vi "SubPanel_Size and Insert.vi"(6 "Border Spacing":i32=-2, 7 "VI":refnum<vi>, 8 "Error":errorcluster, 9 "Frame Ref":refnum<vi>, 10 "Lock Subpanel Size":bool, 11 "Sub Panel":refnum<vi>) -> (0 "Error Out":errorcluster, 1 "Vi Inserted Out":bool, 2 "Success Out":bool, 3 "Sub Panel Out":refnum<vi>)   [LabVIEW 2020]
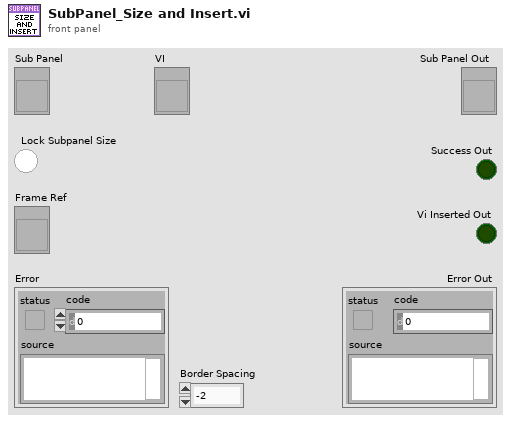
[diagram p1: front panel]
types:
  T1 = typedef "LVRectTypeDef.ctl" = cluster{"Left":i16, "Top":i16, "Right":i16, "Bottom":i16}
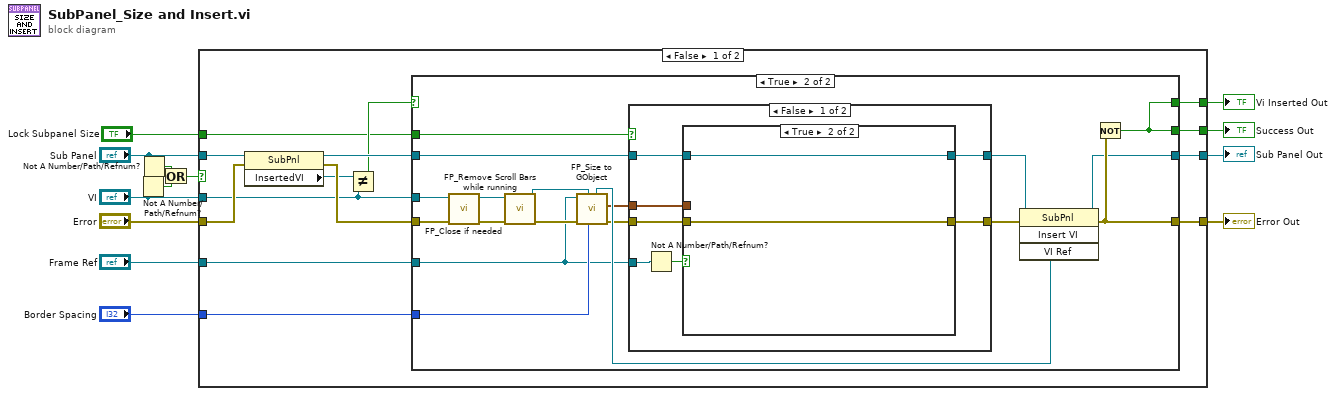
[diagram p0: block diagram]
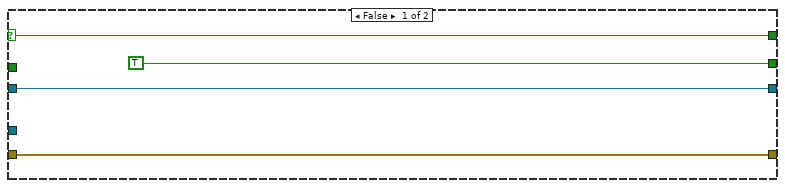
[diagram p2: hidden frame]
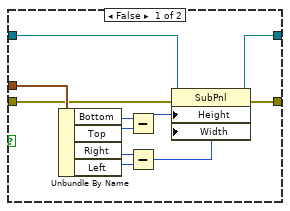
[diagram p3: hidden frame]
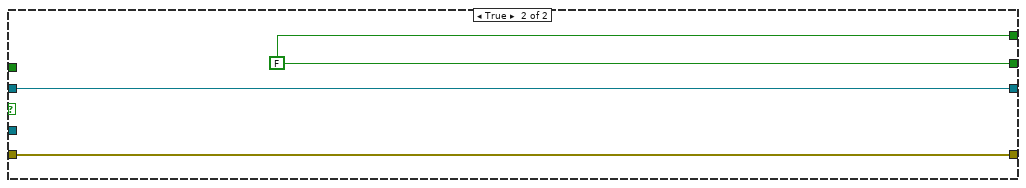
[diagram p5: hidden frame]
diagram:
  n1 = Not A Number/Path/Refnum?(number/path/refnum="VI") -> (NaN/Path/Refnum?=w10:bool)
  n2 = Not A Number/Path/Refnum?(number/path/refnum="Sub Panel") -> (NaN/Path/Refnum?=w11:bool)
  n3 = Or(x=w11, y=w10) -> (x .or. y?=w8:bool)
  n4 = case shown="False" w8 {
    tunnel: [w27 w73] -> w13
    tunnel: "Error" -> [w25 w74]
    tunnel: "Sub Panel" -> [w21 w72]
    tunnel: "VI" -> [w20 _]
    tunnel: [w19 w74] -> w9
    tunnel: [w18 w73] -> w7
    tunnel: "Frame Ref" -> [w17 _]
    tunnel: [w16 w72] -> w5
    tunnel: "Border Spacing" -> [w15 _]
    tunnel: "Lock Subpanel Size" -> [w14 _]
    frame False {
      n5 = property class="SubPnl"(reference=w21, error in=w25) -> (reference out=w26:refnum<vi>, error out=w24:errorcluster, "InsertedVI"=w23:refnum<vi>)
      n6 = Not Equal?(x=w23, y=w20) -> (x != y?=w22:bool)
      n7 = case shown="True" w22 {
        selector: w22 -> [w28 _]
        tunnel: [w30 w47] -> w19
        tunnel: [TRUE w45] -> w27
        tunnel: w26 -> [w29 w46]
        tunnel: w24 -> [w30 w42]
        tunnel: w20 -> [_ w43]
        tunnel: [w28 w45] -> w18
        tunnel: w17 -> [_ w32]
        tunnel: [w29 w44] -> w16
        tunnel: w15 -> [_ w36]
        tunnel: w14 -> [_ w33]
        frame False {
        }
        frame True {
          n8 = call "FP_Close if needed.vi"("Error"=w42, "VI"=w43) -> ("Error Out"=w40:errorcluster, "VI Out"=w41:refnum<vi>)  [unwired: 8 in]
          n9 = call "FP_Remove Scroll Bars while running.vi"("Error"=w40, "VI"=w41) -> ("Error Out"=w37:errorcluster, "VI Out"=w38:refnum<vi>)  [unwired: 8 in]
          n10 = call "FP_Size to GObject.vi"("Border Spacing (2 Px)"=w36, "Calling VI's Ref"=w38, "Error"=w37, "GObj Refnum"=w32) -> ("Error Out"=w34:errorcluster, "Front Panel.PanelBounds Out"=w35:T1, "Calling VI's Ref Out"=w39:refnum<vi>)  [unwired: 2 in, 3 out]
          n11 = case shown="False" w33 {
            tunnel: [w56 w71] -> w49
            tunnel: [w55 w70] -> w48
            tunnel: w46 -> [w54 w70]
            tunnel: w35 -> [w53 _]
            tunnel: w34 -> [w52 w71]
            tunnel: w32 -> [w51 _]
            frame False {
              n12 = Not A Number/Path/Refnum?(number/path/refnum=w51) -> (NaN/Path/Refnum?=w50:bool)
              n13 = case shown="True" w50 {
                tunnel: [w67 w68] -> w56
                tunnel: [w60 w69] -> w55
                tunnel: w54 -> [w59 w69]
                tunnel: w53 -> [w58 _]
                tunnel: w52 -> [w57 w68]
                frame False {
                  n14 = Unbundle By Name(w58) -> ("Bottom"=w61:i16, "Top"=w62:i16, "Right"=w63:i16, "Left"=w64:i16)
                  n15 = Subtract(x=w61, y=w62) -> (x-y=w65:i16)
                  n16 = Subtract(x=w63, y=w64) -> (x-y=w66:i16)
                  n17 = property class="SubPnl"(reference=w59, error in=w57, "Height"=w65, "Width"=w66) -> (reference out=w60:refnum<vi>, error out=w67:errorcluster)
                }
                frame True {
                }
              }
            }
            frame True {
            }
          }
          n18 = invoke class="SubPnl" method="Insert VI"(reference=w48, error in=w49, "VI Ref"=w39) -> (reference out=w44:refnum<vi>, error out=w47:errorcluster)  [unwired: 1 in, 2 out]
          n19 = Not(x=w47) -> (.not. x?=w45:bool)
        }
      }
    }
    frame True {
      w73 = FALSE
    }
  }
  "Success Out" <- w13
  "Error Out" <- w9
  "Vi Inserted Out" <- w7
  "Sub Panel Out" <- w5
